vi "Extract Setpoints from Test Step.vi"(8 "error in (no error)":errorcluster, 11 "Programmer Step":T2) -> (0 "error out":errorcluster, 3 "Data or Setpoints":T1)   [LabVIEW 2012]
uses:
  Data Types/Programmer Step.ctl
  Data Types/Programmer Step References.ctl
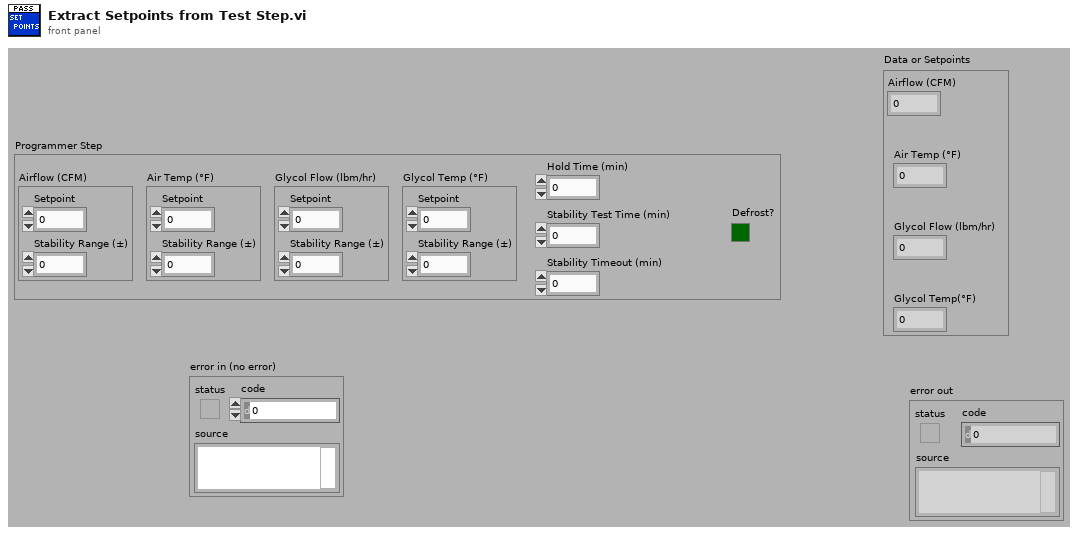
[diagram p1: front panel]
types:
  T1 = cluster{"Airflow (CFM)":dbl, "Air Temp (°F)":dbl, "Glycol Flow (lbm/hr)":dbl, "Glycol Temp(°F)":dbl}
  T2 = typedef "Programmer Step.ctl" = cluster{"Airflow (CFM)":T3, "Air Temp (°F)":T3, "Glycol Flow (lbm/hr)":T3, "Glycol Temp (°F)":T3, "Hold Time (min)":dbl, "Stability Test Time (min)":dbl, "Stability Timeout (min)":dbl, "Defrost?":bool}
  T3 = typedef "Programmer Step References.ctl" = cluster{"Setpoint":dbl, "Stability Range (±)":dbl}
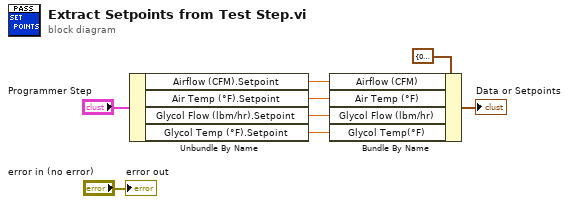
[diagram p0: block diagram]
diagram:
  n1 = Unbundle By Name("Programmer Step") -> ("Airflow (CFM).Setpoint"=w6:dbl, "Air Temp (°F).Setpoint"=w5:dbl, "Glycol Flow (lbm/hr).Setpoint"=w4:dbl, "Glycol Temp (°F).Setpoint"=w3:dbl)
  n2 = Bundle By Name(cluster=T1 {"Airflow (CFM)"=0.0, "Air Temp (°F)"=0.0, "Glycol Flow (lbm/hr)"=0.0, "Glycol Temp(°F)"=0.0} ("Data or Setpoints"), "Airflow (CFM)"=w6, "Air Temp (°F)"=w5, "Glycol Flow (lbm/hr)"=w4, "Glycol Temp(°F)"=w3) -> (→"Data or Setpoints":T1)
  "error out" <- "error in (no error)"
